vi "testEOLsInString.vi"(8 "error in (no error)":errorcluster, 11 "reference in":refnum<class "EasyXMLTest.lvclass">) -> (0 "error out":errorcluster, 3 "reference in":refnum<class "EasyXMLTest.lvclass">)   [LabVIEW 2011, in "EasyXMLTest.lvclass"]
uses:
  EasyXMLTest.lvclass
panel:
  in  "XML String":string="<EmbeddedXML>\r\n  <XMLString>hello\nworld</XMLString>\r\n</EmbeddedXML>"
  in  "EmbeddedXML":cluster{"XMLString":string}={"XMLString"="hello\nworld"}
  out "Produced Data":cluster{"XMLString":string}
  out "Generated XML String":string
  # "Note useage of \\n in data vs \\r\\n in XML entity line delimiters"
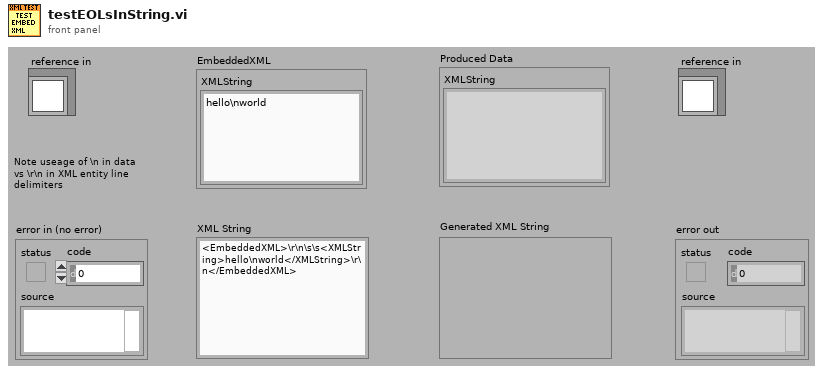
[diagram p1: front panel]
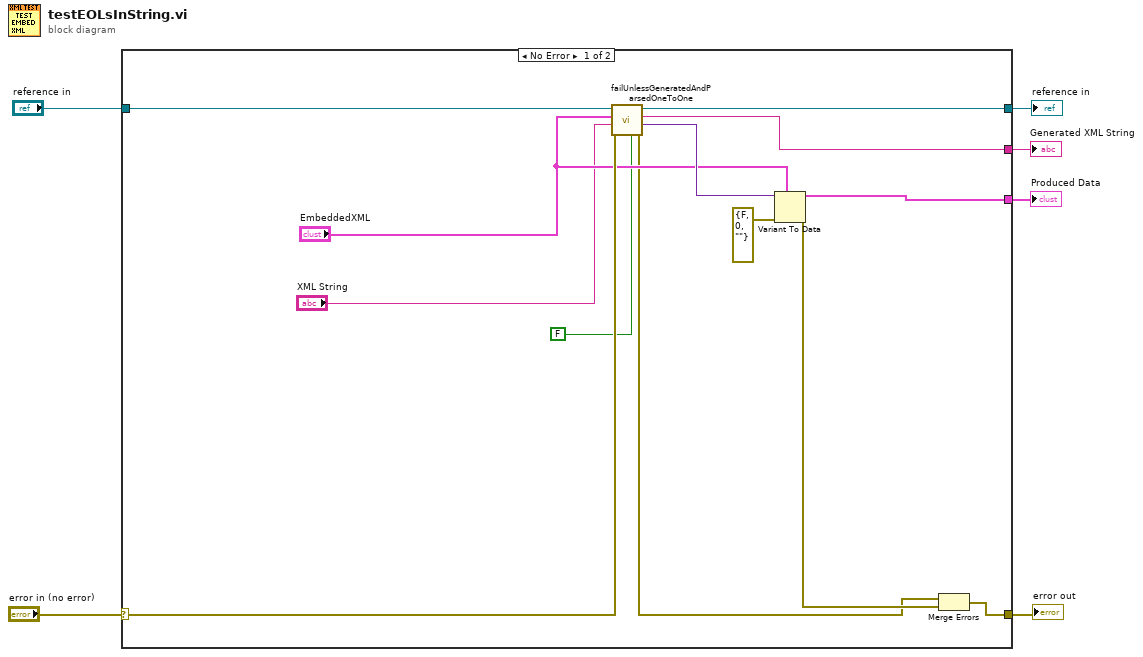
[diagram p0: block diagram]
diagram:
  n1 = case shown="No Error" "error in (no error)" {
    selector: "error in (no error)" -> [w14 w21]
    tunnel: [w19 w21] -> w5
    tunnel: [w16 w20] -> w3
    tunnel: "reference in" -> [w17 w20]
    tunnel: [w15 _] -> w2
    tunnel: [w18 _] -> w1
    frame No Error {
      n2 = call "failUnlessGeneratedAndParsedOneToOne.vi"("Convert EOL? (TRUE)"=FALSE, "error in"=w14, "XML String"="XML String", "Data"="EmbeddedXML", "EasyXMLTest in"=w17) -> ("error out"=w8:errorcluster, "Produced Data"=w11:variant, "Generated XML String"=w15:string, "EasyXMLTest out"=w16:refnum<class "EasyXMLTest.lvclass">)  [unwired: 3 in]
      n3 = Variant To Data(error in=errorcluster {"status"=FALSE, "code"=0, "source"=""}, type="EmbeddedXML", Variant=w11) -> (data=w18:cluster{"XMLString":string}, error out=w13:errorcluster)
      n4 = Merge Errors(w8, w13) -> (w19:errorcluster)
    }
    frame Error {
    }
  }
  "error out" <- w5
  "reference in" <- w3
  "Generated XML String" <- w2
  "Produced Data" <- w1
